vi "Signal_Source_Switch(S4).vi"(8 "error in":errorcluster, 10 "Output":T2(ring), 11 "Input":T1(ring)) -> (0 "error out":errorcluster, 2 "Verfied":bool, 3 "Switches":string)   [LabVIEW 2012]
panel:
  # "Signal Source Switch (S4)"
  # "Switch Input"
  # "Switch Output"
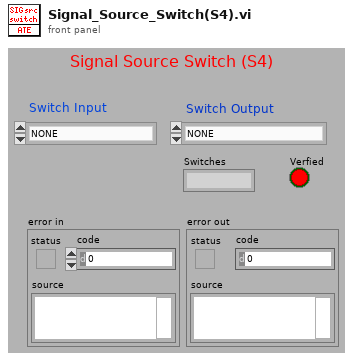
[diagram p1: front panel]
types:
  T1 = enum16{"NONE", "Delay Device", "Signal Generator (J7)", "Inside Noise Box NF (J5)", "2W Term (TM3)"}
  T2 = enum16{"NONE", "Amp Bypass Switch", "Test Pulse Generator", "Power Meter Switch (S5)"}
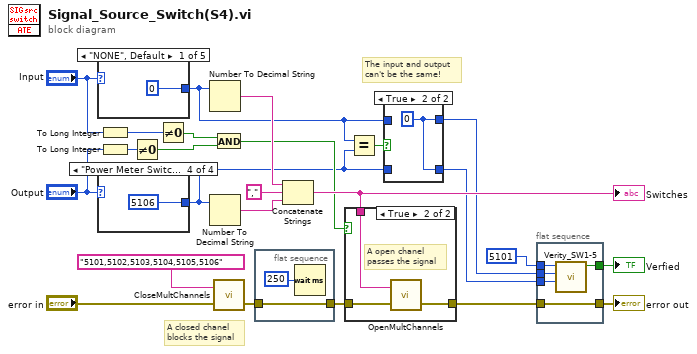
[diagram p0: block diagram]
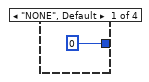
[diagram p3: hidden frame]
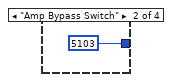
[diagram p4: hidden frame]
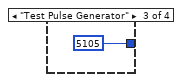
[diagram p5: hidden frame]
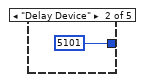
[diagram p6: hidden frame]
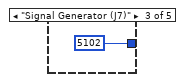
[diagram p7: hidden frame]
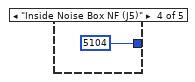
[diagram p8: hidden frame]
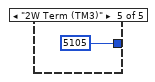
[diagram p9: hidden frame]
diagram:
  # "The input and output\ncan't be the same!"
  # "A closed chanel\nblocks the signal"
  n1 = case shown="\"NONE\", Default" "Input" {
    tunnel: [0 ("Switch ID") 5101 ("Switch ID") 5102 ("Switch ID") 5104 ("Switch ID") 5105 ("Switch ID")] -> w2
    frame "NONE", Default {
    }
    frame "Delay Device" {
    }
    frame "Signal Generator (J7)" {
    }
    frame "Inside Noise Box NF (J5)" {
    }
    frame "2W Term (TM3)" {
    }
  }
  n2 = case shown="\"Power Meter Switch (S5)\\00\"" "Output" {
    tunnel: [0 ("Switch ID") 5103 ("Switch ID") 5105 ("Switch ID") 5106 ("Switch ID")] -> w3
    frame "NONE", Default {
    }
    frame "Amp Bypass Switch" {
    }
    frame "Test Pulse Generator" {
    }
    frame "Power Meter Switch (S5)" {
    }
  }
  n3 = To Long Integer(number="Input") -> (32bit integer=w15:i32)
  n4 = To Long Integer(number="Output") -> (32bit integer=w14:i32)
  n5 = Not Equal To 0?(x=w14) -> (x != 0?=w13:bool)
  n6 = Not Equal To 0?(x=w15) -> (x != 0?=w12:bool)
  n7 = Number To Decimal String(number=w2) -> (decimal integer string=w17:string)  [unwired: 1 in]
  n8 = Number To Decimal String(number=w3) -> (decimal integer string=w18:string)  [unwired: 1 in]
  n9 = And(x=w12, y=w13) -> (x .and. y?=w11:bool)
  n10 = call "CloseMultChannels.vi"("error in (no error)"="error in", "Channels to be closed"="5101,5102,5103,5104,5105,5106" ("Channels to be opened")) -> ("error out"=w20:errorcluster)  [unwired: 1 in]
  n11 = flat-sequence {
    tunnel: w20 -> [w34]
    tunnel: [w34] -> w19
    frame #0 {
      n12 = Wait (ms)(milliseconds to wait=u32 250) -> ()  [unwired: 1 out]
    }
  }
  n13 = Concatenate Strings(w17, ",", w18) -> (w21:string)
  "Switches" <- w21
  n14 = case shown="True" w11 {
    tunnel: w19 -> [w36 w38]
    tunnel: w21 -> [_ w39]
    tunnel: [w36 w37] -> w7
    frame False {
    }
    frame True {
      # "A open chanel\npasses the signal"
      n15 = call "OpenMultChannels.vi"("error in (no error)"=w38, "Channels to be opened"=w39) -> ("error out"=w37:errorcluster)  [unwired: 1 in]
    }
  }
  n16 = Equal?(x=w2, y=w3) -> (x = y?=w10:bool)
  n17 = case shown="True" w10 {
    tunnel: w3 -> [w40 _]
    tunnel: [w40 w42] -> w5
    tunnel: w2 -> [w41 _]
    tunnel: [w41 w42] -> w4
    frame False {
    }
    frame True {
      w42 = 0 ("Switch ID")
    }
  }
  n18 = flat-sequence {
    tunnel: 5101 ("Switch ID") -> [w47]
    tunnel: w4 -> [w46]
    tunnel: w5 -> [w45]
    tunnel: [w44] -> w9
    tunnel: w7 -> [w43]
    tunnel: [w43] -> w6
    frame #0 {
      n19 = call "Verity_SW1-5.vi"("Output Switch ID"=w45, "Input Switch ID"=w46, "Base Switch ID"=w47) -> ("Verfied"=w44:bool)  [unwired: 7 in, 1 out]
    }
  }
  "error out" <- w6
  "Verfied" <- w9
